vi "Init Node Info.vi"(8 "error in (no error)":errorcluster, 11 "DiscoveryService in":refnum<class "DiscoveryService.lvclass">) -> (0 "error out":errorcluster, 3 "DiscoveryService out":refnum<class "DiscoveryService.lvclass">)   [LabVIEW 2020, in "Vecto.lvlib" / "DiscoveryService.lvclass"]
uses:
  DiscoveryService.lvclass
  proto/Discovery/Data.ctl
  proto/Service/Data.ctl
  proto/ServiceType/Enumeration.ctl
  DiscoveryService.lvclass/DiscoveryService.ctl
  Node Config/Node Config.lvclass/Node Config.ctl
  proto/Discovery/Class/Msg.lvclass/Msg.ctl
  proto/Discovery/Class/Msg.lvclass
  proto/ServiceType/ServiceType.lvlib
  proto/Service/Service.lvlib
  proto/Discovery/Discovery.lvlib
  Node Config/Node Config.lvclass
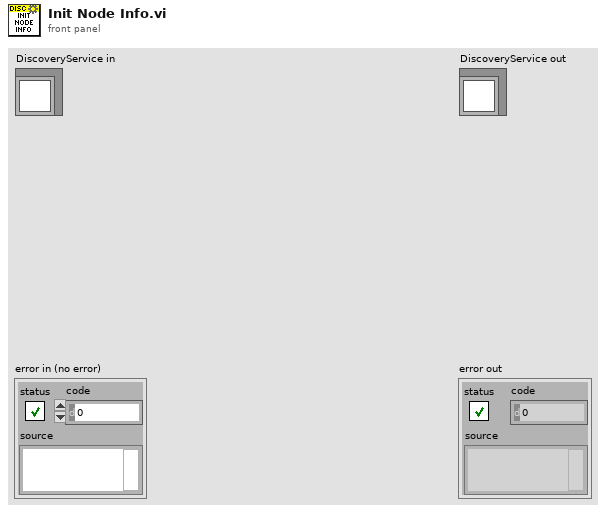
[diagram p1: front panel]
types:
  T1 = typedef "Discovery.lvlib/Data.ctl" = cluster{"node_id":u32, "name":string, "ip":u32, "status":string, "services":T2[], "system":string, "cluster":string}
  T2 = typedef "Service.lvlib/Data.ctl" = cluster{"type":T3, "port":i32}
  T3 = typedef "ServiceType.lvlib/Enumeration.ctl" = enum16{"SERVICETYPE_UNKNOWN", "SERVICETYPE_TCPSERVER", "SERVICETYPE_HTTPSERVER"}
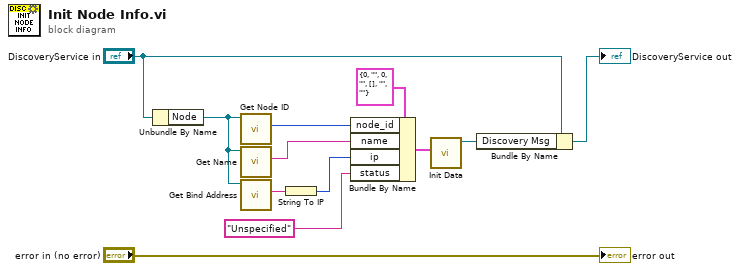
[diagram p0: block diagram]
diagram:
  n1 = Unbundle By Name("DiscoveryService in") -> ("Node"=w4:refnum<class "Node Config.lvclass">)
  n2 = call "Get Node ID.vi"("Node in"=w4) -> ("Node ID"=w11:u32)  [unwired: 8 in, 2 out]
  n3 = call "Get Name.vi"("Node in"=w4) -> ("Name"=w10:string)  [unwired: 8 in, 2 out]
  n4 = call "Get Bind Address.vi"("Node in"=w4) -> ("Bind Address"=w3:string)  [unwired: 8 in, 2 out]
  n5 = String To IP(1:w3) -> (0:w2:u32)
  n6 = Bundle By Name(cluster=T1 {"node_id"=0, "name"="", "ip"=0, "status"="", "services"=[], "system"="", "cluster"=""} ("Discovery"), "node_id"=w11, "name"=w10, "ip"=w2, "status"="Unspecified") -> (w8:T1)
  n7 = call "Init Data.vi"("Data"=w8) -> ("Msg out"=w6:refnum<class "Msg.lvclass">)  [unwired: 10 in]
  n8 = Bundle By Name(cluster="DiscoveryService in", "Discovery Msg"=w6) -> (→"DiscoveryService out":refnum<class "DiscoveryService.lvclass">)
  "error out" <- "error in (no error)"
